vi "IS PolyVI Instance DBL To JSON Cluster .vi"(3 "Stream Time (optional)":timestamp=timestamp(1451714400 s since 1904-01-01), 4 "Stream Value":dbl, 5 "Stream Key":string) -> (1 "JSON Cluster Array out":T1[](array[typedef]))   [LabVIEW 2018]
doc: "This VI is part of a Polymorphic collection of VIs that transform data into an Array of TypeDef Clusters. The Cluster Type-Definition represents the JSON format specific to the Initial State API - which includes a Stream Key, a data value, and an epoch time. This particular polymorphic instance takes DBL as input for the data value."
uses:
  Controls/IS Data Point TypeDef (String).ctl
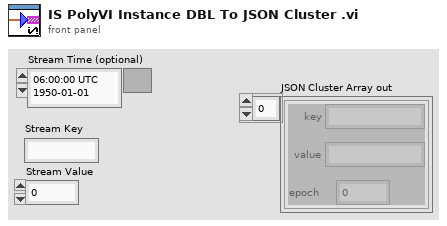
[diagram p1: front panel]
types:
  T1 = typedef "IS Data Point TypeDef (String).ctl" = cluster{"key":string, "value":string, "epoch":dbl}
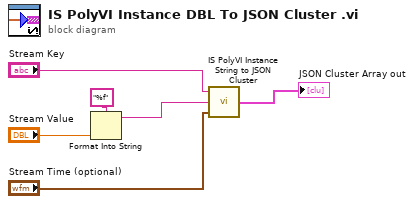
[diagram p0: block diagram]
diagram:
  n1 = Format Into String(format string="%f", "Stream Value") -> (resulting string=w3:string)  [unwired: 2 in, 1 out]
  n2 = call "IS PolyVI Instance String to JSON Cluster.vi"("Stream Time (optional)"="Stream Time (optional)", "Stream Value"=w3, "Stream Key"="Stream Key") -> ("JSON Cluster Array out"=→"JSON Cluster Array out":T1[])  [unwired: 2 in]
